vi "Remove outliars before calculations.vi"(3 "Pressure IN":dbl[](array[numeric])=[155.29465785925402, 148.65463937715, 142.579196662662, 136.74673592411, 130.898195495974, 126.09394157471002, 121.39956553227, 116.56761881227801, 111.924161786854, 107.903346074766, 103.852157615686, 99.661611846878, 95.85340536373401, 92.392698838822, 89.05169666970201, 86.22256461900601, 83.517603504542, 80.93681332631, 77.781620903494, 75.232096788342, 72.814783454214, 70.33404467783801, 68.057875285614, 67.562978172862, 66.17119170775801, 63.98971382086201, 63.526976087278, 61.977072674598006, 60.04215002799001, 57.842805819334004, 57.47475959107801], 4 "Peak Pressure IN":dbl[](array[numeric])=[0.07771849965598676, 0.12149098796797375, 0.22243570591200523, 0.450231308351988, 0.4984703771039847, 0.7110796060480027, 0.9567415302479958, 1.2122299314160045, 1.4069728385999838, 1.7893121242639864, 2.1412786629359886, 2.0769599046000025, 2.2297169556480156, 2.4342863397999963, 2.4369662880640135, 2.71568090752001, 3.0024353717679872, 2.955089619104001, 2.1752246742799883, 2.315475300095997, 2.1269856055279917, 1.848270986071995, 1.5436502000639933, 0.012506425232004403, 1.6419149697440076, 1.3471206607040074, 0.014293057407996912, 1.2318828853520074, 1.2962016436880077, 1.1318314834960006, 0.00982647696801564], 5 "Pulse Rate IN":dbl[](array[numeric])=[57.25190839694656, 57.08848715509039, 55.60704355885079, 56.12722170252573, 58.53658536585366, 58.30903790087464, 53.19148936170213, 55.65862708719851, 57.03422053231939, 54.74452554744525, 53.57142857142857, 55.65862708719851, 55.29953917050691, 54.29864253393665, 55.71030640668524, 55.81395348837209, 55.65862708719851, 54.44646098003629, 56.12722170252573, 56.444026340545626, 54.54545454545454, 55.147058823529406, 178.04154302670622, 81.52173913043478, 54.005400540054005, 178.04154302670622, 82.53094910591471, 56.17977528089887, 54.794520547945204, 170.94017094017096]) -> (0 "Pressure OUT":dbl[](array[numeric])=[57.47475959107801], 1 "Peak Pressure OUT":dbl[](array[numeric])=[0.00982647696801564], 2 "Pulse Rate OUT":dbl[](array[numeric]))   [LabVIEW 2017]
doc: "[Covers: AlgorithmReq2]"
uses:
  <vilib>/Analysis/baseanly.llb/Mean (DBL).vi
  <vilib>/Analysis/NI_AALBase.lvlib
panel:
  # "Outputs"
  # "Inputs"
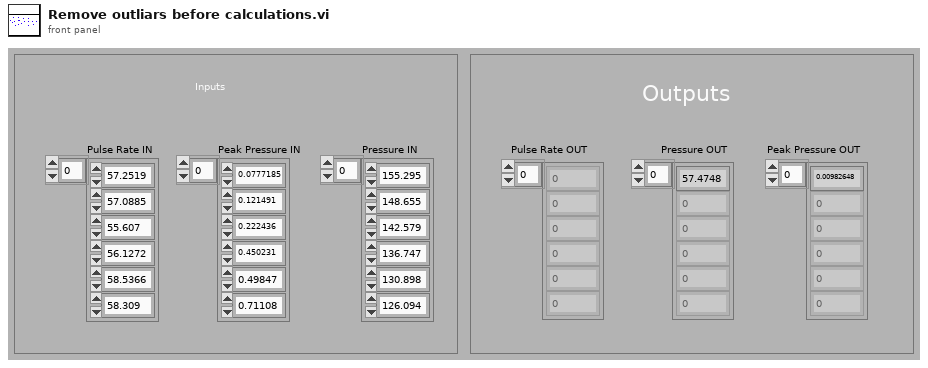
[diagram p1: front panel]
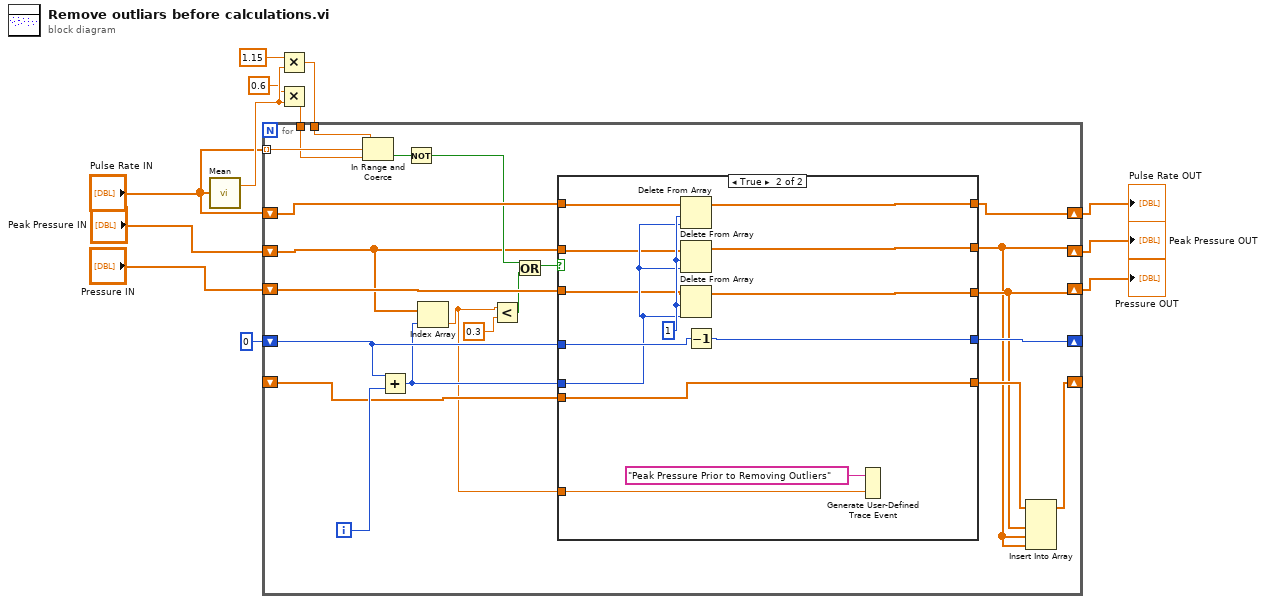
[diagram p0: block diagram]
diagram:
  n1 = call-poly <vilib>:"Mean.vi"("X"="Pulse Rate IN") -> ("mean"=w8:dbl)  [unwired: 1 out]
  n2 = Multiply(x=1.15, y=w8) -> (x*y=w11:dbl)
  n3 = Multiply(x=0.6, y=w8) -> (x*y=w10:dbl)
  n4 = for {
    shift-right: [w32] -> w7
    shift-left: "Pulse Rate IN" -> [w33]
    shift-right: [w14] -> w4
    shift-left: "Peak Pressure IN" -> [w21]
    shift-right: [w15] -> w3
    shift-left: "Pressure IN" -> [w26]
    tunnel: "Pulse Rate IN" -> [w34] mode=indexing
    tunnel: w10 -> [w31]
    tunnel: w11 -> [w30]
    shift-right: [w29] -> _
    shift-left: 0 -> [w27]
    shift-right: [w16] -> _
    shift-left: _ -> [w18]
    i -> [w28]
    n5 = In Range and Coerce(upper limit=w30, x=w34, lower limit=w31) -> (In Range?=w23:bool)  [unwired: 1 out]
    n6 = Add(x=w27, y=w28) -> (x+y=w25:i32)
    n7 = Not(x=w23) -> (.not. x?=w22:bool)
    n8 = Index Array(array=w21, index=w25) -> (element=w13:dbl)
    n9 = Less?(x=w13, y=0.3 ("x")) -> (x < y?=w19:bool)
    n10 = Or(x=w22, y=w19) -> (x .or. y?=w24:bool)
    n11 = case shown="True" w24 {
      tunnel: w33 -> [w39 w43]
      tunnel: w21 -> [w38 w44]
      tunnel: w26 -> [w37 w45]
      tunnel: [w39 w52] -> w32
      tunnel: [w38 w51] -> w14
      tunnel: [w37 w50] -> w15
      tunnel: w27 -> [w36 w47]
      tunnel: [w36 w48] -> w29
      tunnel: w25 -> [_ w46]
      tunnel: [w35 w42] -> w17
      tunnel: w18 -> [w35 w42]
      tunnel: w13 -> [_ w41]
      frame False {
      }
      frame True {
        w49 = 1 ("length")
        n12 = Delete From Array(array=w43, length=w49, index=w46) -> (array with subset deleted=w52:dbl[])  [unwired: 1 out]
        n13 = Delete From Array(array=w44, length=w49, index=w46) -> (array with subset deleted=w51:dbl[])  [unwired: 1 out]
        n14 = Delete From Array(array=w45, length=w49, index=w46) -> (array with subset deleted=w50:dbl[])  [unwired: 1 out]
        n15 = Decrement(x=w47) -> (x-1=w48:i32)
        n16 = Generate User-Defined Trace Event(1:w41, 2:"Peak Pressure Prior to Removing Outliers" ("trace string")) -> ()
      }
    }
    n17 = Insert Into Array(array=w17, new element #1=w15, new element #2=w14, new element #3=w14) -> (w16:dbl[])  [unwired: 1 in]
  }
  "Pulse Rate OUT" <- w7
  "Peak Pressure OUT" <- w4
  "Pressure OUT" <- w3
